vi "Optimal FIR Filter - DFD.vi"() -> ()   [LabVIEW 2023]
doc: "Demonstrates how to solve for an optimal FIR filter using VIs in the LabVIEW Digital Filter Design Toolkit."
uses:
  <vilib>/addons/Digital Filter Design/Analysis.llb/DFD Plot Freq Response (Linear-Spaced).vi
  <vilib>/Analysis/NI_AALBase.lvlib
  <vilib>/addons/Digital Filter Design/NI_DigFilterLicensed.lvlib
panel:
  in  "Band Parameters":T1(array[cluster])=[{"Amplitude"=2.0, "Lower Freq"=0.0, "Higher Freq"=0.1, "Weighted\nRipple"=1.0}, {"Amplitude"=0.0, "Lower Freq"=0.2, "Higher Freq"=0.25, "Weighted\nRipple"=1.0}, {"Amplitude"=1.0, "Lower Freq"=0.3, "Higher Freq"=0.5, "Weighted\nRipple"=1.0}] {"Amplitude" min=0.0 format="%0.2f"; "Lower Freq" format="%0.2f"; "Higher Freq" format="%0.2f"; "Weighted\nRipple" format="%0.2e"}
  in  "stop":bool
  in  "stop copy":bool
  in  "order":i32=9
  out "Magnitude Response":cluster{"f0":dbl, "df":dbl, "values":dbl[]}[](graph)
  # "Select Help»Show Context Help and move the cursor over the VI icon for more information."
  # "Optimal FIR Filter Design"
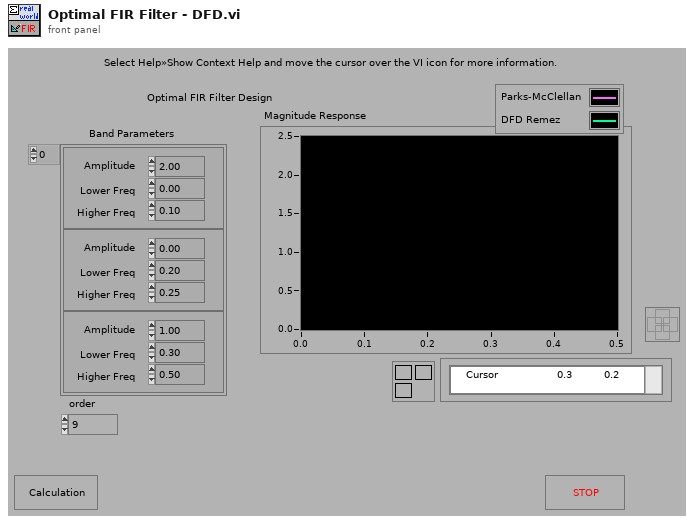
[diagram p1: front panel]
types:
  T1 = cluster{"Amplitude":dbl, "Lower Freq":dbl, "Higher Freq":dbl, "Weighted\nRipple":dbl}[]
  T2 = cluster{"Lower Freq":dbl, "Amplitude":dbl, "Weighted\nRipple":dbl}
  T3 = cluster{"Higher Freq":dbl, "Amplitude":dbl, "Weighted\nRipple":dbl}
  T4 = cluster{"Higher Freq":dbl, "Amplitude":dbl, "Weighted\nRipple":dbl}[]
  T5 = cluster{cluster{"Higher Freq":dbl, "Amplitude":dbl, "Weighted\nRipple":dbl}[], dbl}
  T6 = typedef "NI_DigFilterLicensed.lvlib/DFD Filter Obj.ctl" = cluster{"mSRate_Fs":dbl, "mSRate_Version":string, "mSRate_Comments":string, "mSRate_OrgCoef":T7, "mSRate_CurCoef":T7, "mSRate_Quantized?":bool, "mSRate_QCoef":T7, "mSRate_QSettings":T9[], "mSRate_Order":i32, "mSRate_Scaling":cluster{"mSRate_ScaleByPowerOf2?":bool, "mSRate_ScaleType":T11}}
  T7 = typedef "NI_DigFilterLicensed.lvlib/DFD Filter Coef.ctl" = cluster{"type":T8, "gain":dbl, "coef a (k)":dbl[], "coef b (v)":dbl[]}
  T8 = typedef "NI_DigFilterLicensed.lvlib/DFD Filter Structure Type Selector.ctl" = enum16{"Undefined", "FIR Direct Form", "FIR Direct Form Transposed", "FIR Symmetric", "FIR Antisymmetric", "IIR Direct Form I", "IIR Direct Form I Transposed", "IIR Direct Form II", "IIR Direct Form II Transposed", "IIR Cascaded Second Order Sections Form I", "IIR Cascaded Second Order Sections Form I Transposed", "IIR Cascaded Second Order Sections Form II", "IIR Cascaded Second Order Sections Form II Transposed", "Lattice Allpass (basic sections)", "Lattice Allpass (one multiplier sections)", "Lattice Allpass (normalized sections)", "Lattice AR (basic sections)", "Lattice AR (one multiplier sections)", "Lattice AR (normalized sections)", "Lattice MA (minimum phase)", "Lattice MA (maximum phase)", "Lattice ARMA (basic sections)", "Lattice ARMA (one multiplier sections)", "Lattice ARMA (normalized sections)"}
  T9 = typedef "NI_DigFilterLicensed.lvlib/dfd_Internal Quantization Settings.ctl" = cluster{"source":T10, "wl":i16, "iwl":i16, "overflow mode":enum16{"Saturation", "Wrap"}, "rounding mode":enum16{"Nearest", "Truncation"}, "signed?":bool}
  T10 = typedef "NI_DigFilterLicensed.lvlib/dfd_Internal Quantization Srcs.ctl" = u16
  T11 = typedef "NI_DigFilterLicensed.lvlib/DFD Coef Norm Type.ctl" = enum16{"No Norm", "Time Domain 1-Norm", "Time Domain 2-Norm", "Time Domain Inf-Norm"}
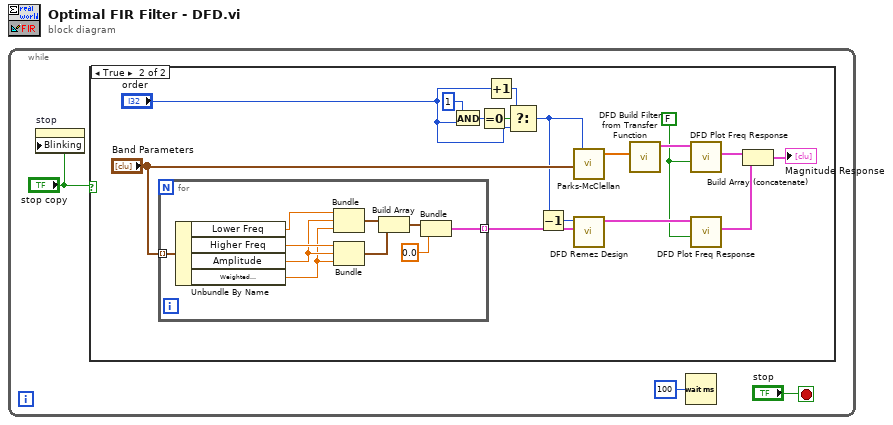
[diagram p0: block diagram]
diagram:
  n1 = while {
    stop <- "stop" stop-if-true
    n2 = property on="stop" class="Bool"("Blinking"="stop copy") -> ()  [unwired: 2 in, 2 out]
    n3 = case shown="True" "stop copy" {
      frame False {
      }
      frame True {
        w7 = FALSE
        n4 = for {
          tunnel: "Band Parameters" -> [w29] mode=indexing
          tunnel: [w20] -> w13 mode=indexing
          n5 = Unbundle By Name(w29) -> ("Lower Freq"=w28:dbl, "Higher Freq"=w27:dbl, "Amplitude"=w26:dbl, "Weighted\nRipple"=w25:dbl)
          n6 = Bundle("Lower Freq"=w28, "Amplitude"=w26, "Weighted\nRipple"=w25) -> (w24:T2)  [unwired: 1 out]
          n7 = Bundle("Higher Freq"=w27, "Amplitude"=w26, "Weighted\nRipple"=w25) -> (w23:T3)  [unwired: 1 out]
          n8 = Build Array(w24, w23) -> (w22:T4)
          n9 = Bundle(w22, 0.0) -> (w20:T5)  [unwired: 1 out]
        }
        n10 = And(x=1, y="order") -> (x .and. y?=w17:i32)
        n11 = Equal To 0?(x=w17) -> (x = 0?=w16:bool)
        n12 = Increment(x="order") -> (x+1=w15:i32)
        n13 = Select(t=w15, s=w16, f="order") -> (s? t:f=w11:i32)
        n14 = Decrement(x=w11) -> (x-1=w12:i32)
        n15 = call <vilib>:"Parks-McClellan.vi"("Band Parameters"="Band Parameters", "# of taps"=w11) -> ("h"=w10:dbl[])  [unwired: 2 in, 2 out]
        n16 = call <vilib>:"DFD Remez Design.vi"("band specs"=w13, "order"=w12) -> ("filter out"=w8:T6)  [unwired: 5 in, 4 out]
        n17 = call <vilib>:"DFD Build Filter from Transfer Function.vi"("numerator"=w10) -> ("filter out"=w9:T6)  [unwired: 3 in, 7 out]
        n18 = call-poly <vilib>:"DFD Plot Freq Response.vi"("dB on? (T)"=w7, "filter in"=w9) -> ("magnitude response"=w6:cluster{"f0":dbl, "df":dbl, "values":dbl[]}[])  [unwired: 6 in, 3 out]
        n19 = call-poly <vilib>:"DFD Plot Freq Response.vi"("dB on? (T)"=w7, "filter in"=w8) -> ("magnitude response"=w5:cluster{"f0":dbl, "df":dbl, "values":dbl[]}[])  [unwired: 6 in, 3 out]
        n20 = Build Array (concatenate)(w6, w5) -> (→"Magnitude Response":cluster{"f0":dbl, "df":dbl, "values":dbl[]}[])
      }
    }
    n21 = Wait (ms)(milliseconds to wait=u32 100) -> ()  [unwired: 1 out]
  }
